vi "update_SS_plots.vi"(6 "other-frd":T1, 7 "freqs-iter":i32, 8 "error in (no error)":errorcluster, 10 "experiment-data":T4, 11 "figures-in":T2) -> (0 "error out":errorcluster, 1 "experiment-data (out)":T4, 2 "FRD-out":T1, 3 "figures-out":T2)   [LabVIEW 2017]
uses:
  auto-sys-id/controls/SS_figures.ctl
  auto-sys-id/controls/bode_figure.ctl
  auto-sys-id/controls/SS_experimental-data.ctl
  auto-sys-id/controls/SS_FourierData.ctl
  auto-sys-id/controls/FrdData.ctl
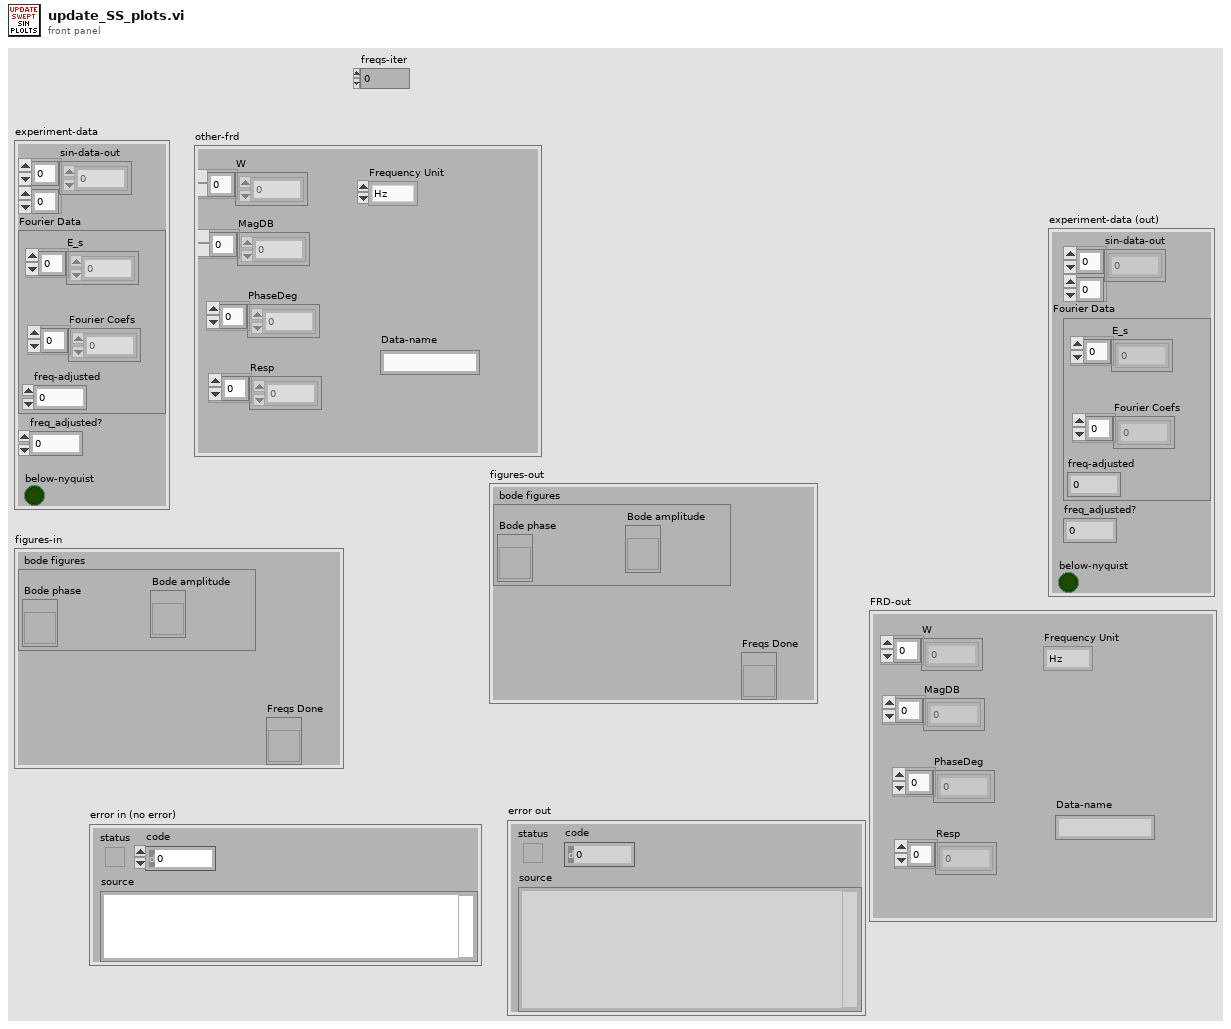
[diagram p1: front panel]
types:
  T1 = typedef "FrdData.ctl" = cluster{"Frequency Unit":enum16{"Hz", "rad/s"}, "W":dbl[], "MagDB":dbl[], "PhaseDeg":dbl[], "Resp":cdb[], "Data-name":string}
  T2 = typedef "SS_figures.ctl" = cluster{"bode figures":T3, "Freqs Done":refnum<vi>}
  T3 = typedef "bode_figure.ctl" = cluster{"Bode phase":refnum<vi>, "Bode amplitude":refnum<vi>}
  T4 = typedef "SS_experimental-data.ctl" = cluster{"sin-data-out":dbl[][], "Fourier Data":T5, "freq_adjusted?":dbl, "below-nyquist":bool}
  T5 = typedef "SS_FourierData.ctl" = cluster{"E_s":dbl[], "Fourier Coefs":cdb[], "freq-adjusted":dbl}
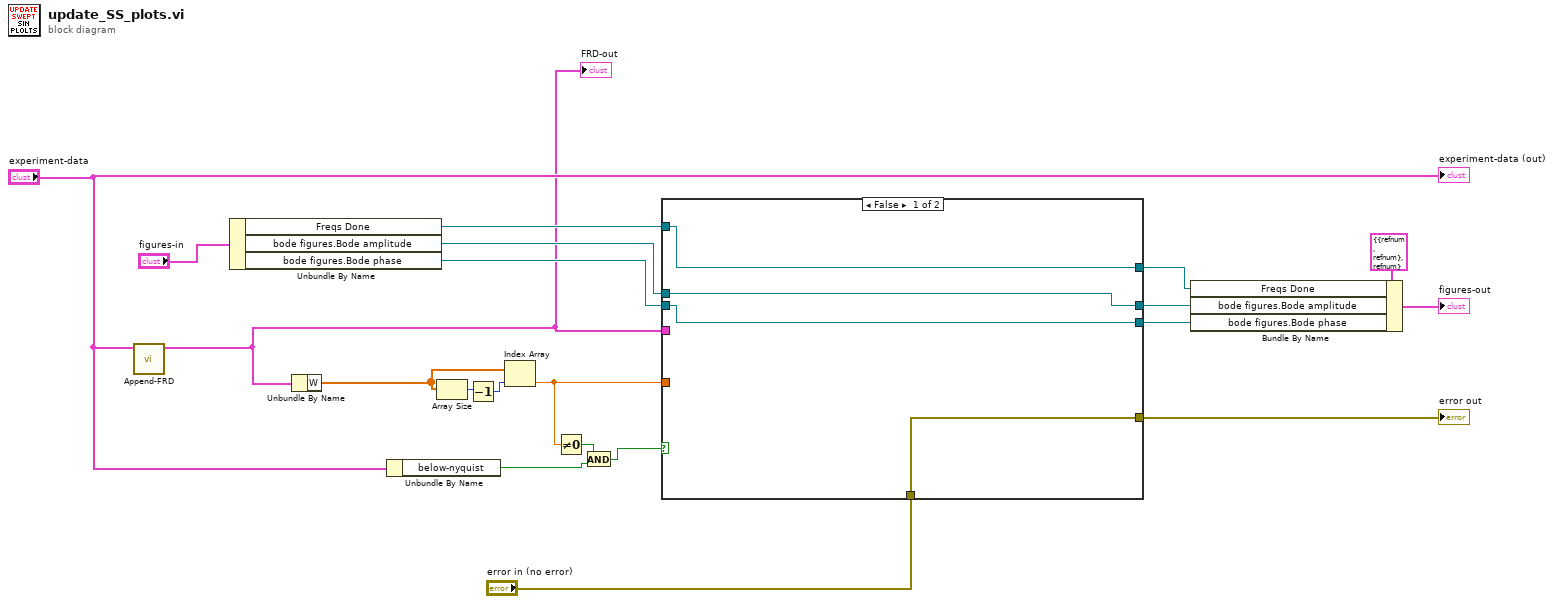
[diagram p0: block diagram]
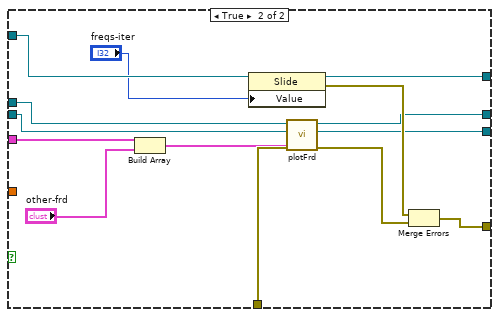
[diagram p2: hidden frame]
diagram:
  n1 = call "Append-FRD.vi"("experiment-data"="experiment-data") -> ("FRD-out"=w7:T1)  [unwired: 10 in]
  "FRD-out" <- w7
  n2 = Unbundle By Name("figures-in") -> ("Freqs Done"=w9:refnum<vi>, "bode figures.Bode amplitude"=w14:refnum<vi>, "bode figures.Bode phase"=w13:refnum<vi>)
  n3 = Unbundle By Name(w7) -> ("W"=w6:dbl[])
  n4 = Unbundle By Name("experiment-data") -> ("below-nyquist"=w10:bool)
  n5 = Array Size(array=w6) -> (size(s)=w19:i32)
  n6 = Decrement(x=w19) -> (x-1=w18:i32)
  n7 = Index Array(array=w6, index=w18) -> (element=w17:dbl)
  n8 = Not Equal To 0?(x=w17) -> (x != 0?=w12:bool)
  n9 = And(x=w12, y=w10) -> (x .and. y?=w11:bool)
  n10 = case shown="False" w11 {
    tunnel: [w24 w37] -> w20
    tunnel: w7 -> [_ w30]
    tunnel: w17 -> [_ _]
    tunnel: w14 -> [w23 w36]
    tunnel: w13 -> [w22 w35]
    tunnel: "error in (no error)" -> [w24 w34]
    tunnel: w9 -> [w21 w33]
    tunnel: [w23 w27] -> w3
    tunnel: [w22 w26] -> w2
    tunnel: [w21 w25] -> w1
    frame False {
    }
    frame True {
      n11 = Build Array(w30, "other-frd") -> (w29:T1[])
      n12 = property class="Slide"(reference=w33, "Value"="freqs-iter") -> (reference out=w25:refnum<vi>, error out=w32:errorcluster)  [unwired: 1 in]
      n13 = call "plotFrd.vi"("error in (no error)"=w34, "FRD-array"=w29, "Phase Graph Reference in"=w35, "Magnitude Graph Reference in"=w36) -> ("error out"=w38:errorcluster, "Phase Graph Reference out"=w26:refnum<vi>, "Magnitude Graph Reference out"=w27:refnum<vi>)  [unwired: 5 in]
      n14 = Merge Errors(w32, w38) -> (w37:errorcluster)
    }
  }
  "error out" <- w20
  n15 = Bundle By Name(cluster=T2 {"bode figures"={"Bode phase"=refnum, "Bode amplitude"=refnum}, "Freqs Done"=refnum} ("figures-out 2"), "Freqs Done"=w1, "bode figures.Bode amplitude"=w3, "bode figures.Bode phase"=w2) -> (→"figures-out":T2)
  "experiment-data (out)" <- "experiment-data"
